vi "Initialize_Angle.vi"(8 "error in (no error)":errorcluster, 10 "Angle.lvclass":refnum<class "Angle.lvclass">, 11 "PolarVector in":refnum<class "PolarVector.lvclass">) -> (0 "error out":errorcluster, 3 "PolarVector out":refnum<class "PolarVector.lvclass">)   [LabVIEW 2011, in "PolarVector.lvclass"]
uses:
  PolarVector.lvclass
  Angles/Angle/Angle.lvclass
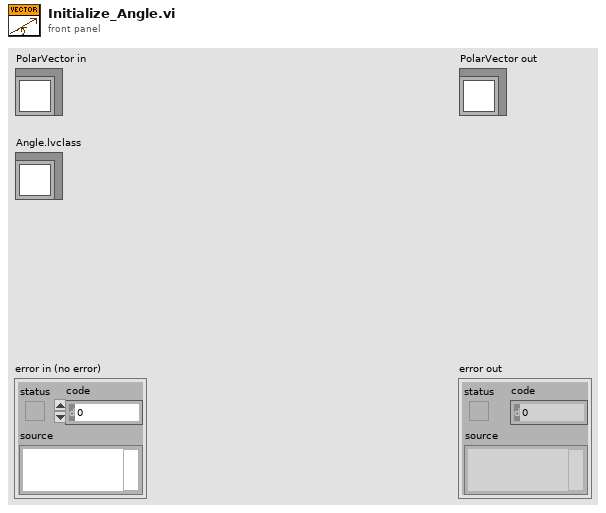
[diagram p1: front panel]
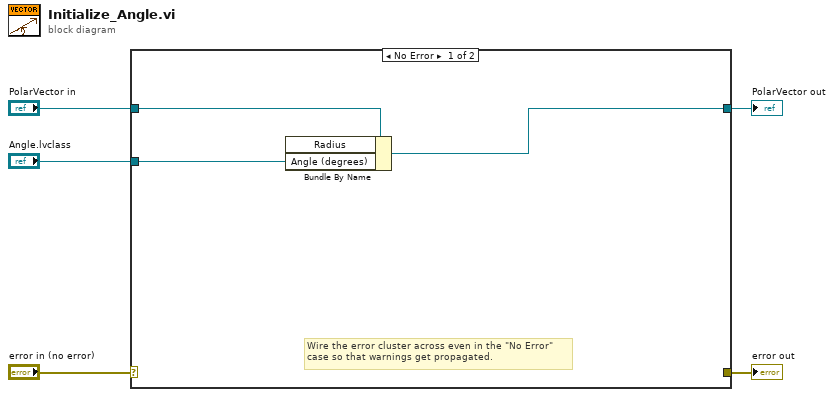
[diagram p0: block diagram]
diagram:
  n1 = case shown="No Error" "error in (no error)" {
    selector: "error in (no error)" -> [_ w10]
    tunnel: [_ w10] -> w4
    tunnel: [w6 w9] -> w2
    tunnel: "PolarVector in" -> [w8 w9]
    tunnel: "Angle.lvclass" -> [w7 _]
    frame No Error {
      # "Wire the error cluster across even in the \"No Error\"\ncase so that warnings get propagated."
      n2 = Bundle By Name(cluster=w8, "Angle (degrees)"=w7) -> (w6:refnum<class "PolarVector.lvclass">)  [unwired: 1 in]
    }
    frame Error {
    }
  }
  "error out" <- w4
  "PolarVector out" <- w2
